vi "MarkerRole.vi"(7 "firstCall":bool, 8 "error in (no error)":errorcluster, 10 "Game in":refnum<class "Game.lvclass">, 11 "MarkerRole in":refnum<class "MarkerRole.lvclass">) -> (0 "error out":errorcluster, 1 "Game out":refnum<class "Game.lvclass">, 2 "Robot out":refnum<class "Robot.lvclass">, 3 "MarkerRole out":refnum<class "MarkerRole.lvclass">)   [LabVIEW 2020, in "MarkerRole.lvclass"]
uses:
  MarkerRole.lvclass
  Tacticbook_class/Tacticbook.lvclass
  MarkerTactic_class/MarkerTactic.lvclass
  MarkerTactic_class/MarkerTacticStates.ctl
  Game_class/Game.lvclass
  Robot_class/Robot.lvclass
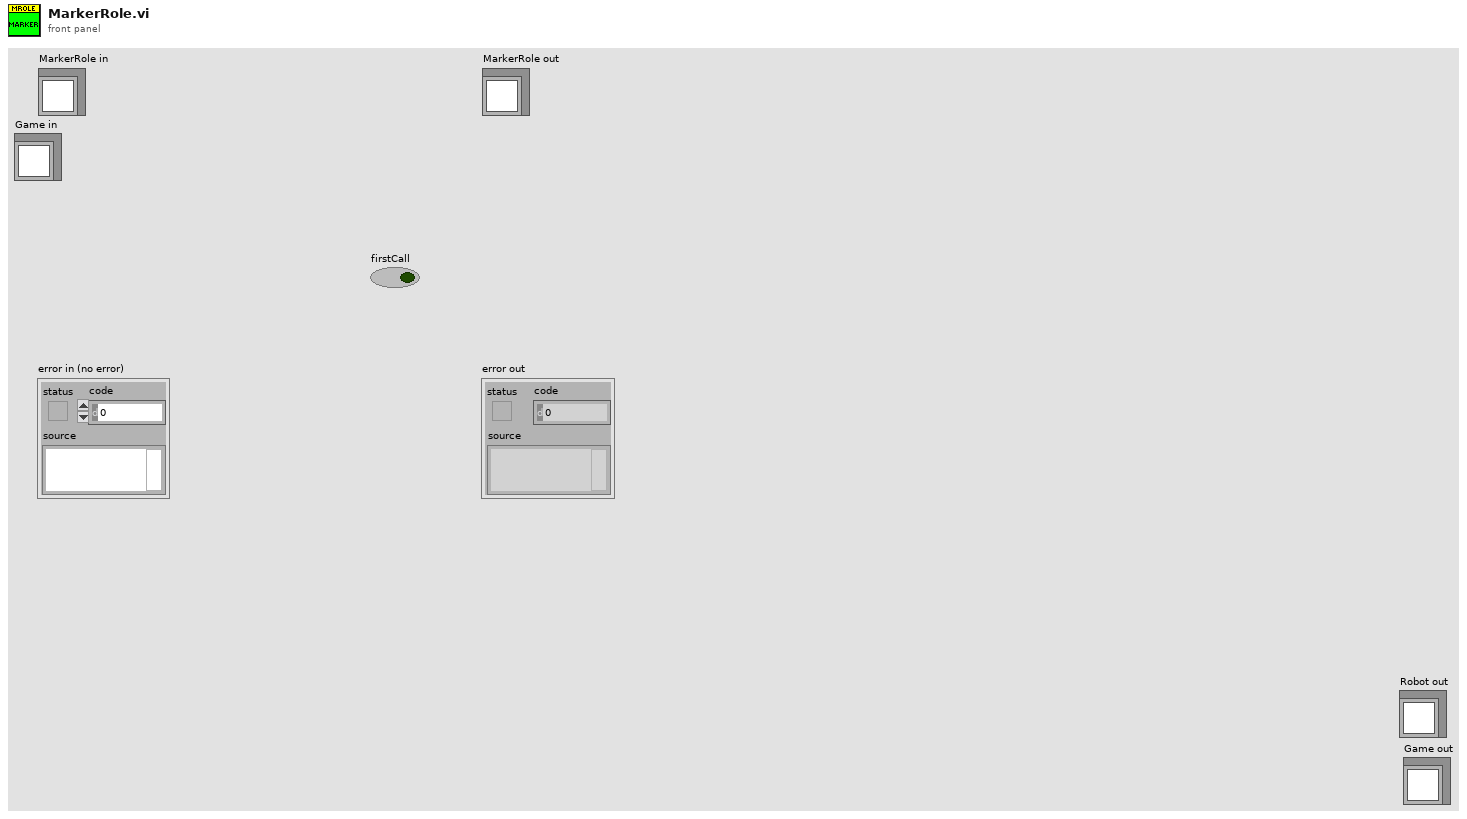
[diagram p1: front panel]
types:
  T1 = typedef "MarkerTacticStates.ctl" = enum16{"Exit", "BlockOurGoal", "FollowAttacker", "BlockEnemyPass"}
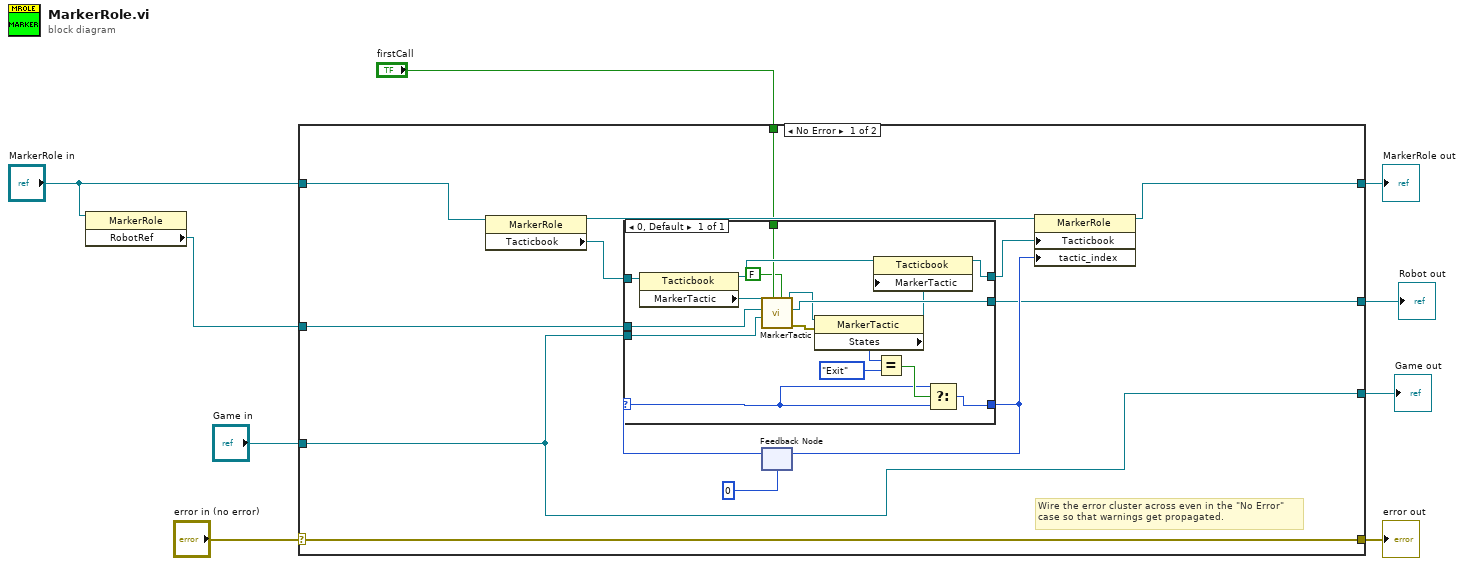
[diagram p0: block diagram]
diagram:
  n1 = property class="MarkerRole"(reference="MarkerRole in") -> ("RobotRef"=w2:refnum<class "Robot.lvclass">)  [unwired: 1 in, 2 out]
  n2 = case shown="No Error" "error in (no error)" {
    selector: "error in (no error)" -> [w22 w42]
    tunnel: [w22 w42] -> w8
    tunnel: [w14 w41] -> w7
    tunnel: "MarkerRole in" -> [w15 w41]
    tunnel: "Game in" -> [w12 w40]
    tunnel: [w13 _] -> w4
    tunnel: [w12 w40] -> w3
    tunnel: w2 -> [w11 _]
    tunnel: "firstCall" -> [w10 _]
    frame No Error {
      # "Wire the error cluster across even in the \"No Error\"\ncase so that warnings get propagated."
      n3 = property class="MarkerRole"(reference=w15) -> (reference out=w21:refnum<class "MarkerRole.lvclass">, "Tacticbook"=w18:refnum<class "Tacticbook.lvclass">)  [unwired: 1 in, 1 out]
      n4 = feedback #1(0) -> (w19:i32)
      n5 = case shown="0, Default" w19 {
        selector: w19 -> [w26]
        tunnel: [w32] -> w17
        tunnel: w18 -> [w39]
        tunnel: [w37] -> w13
        tunnel: [w29] -> w16
        tunnel: w12 -> [w28]
        tunnel: w11 -> [w27]
        tunnel: w10 -> [w24]
        frame 0, Default {
          n6 = property class="Tacticbook"(reference=w39) -> (reference out=w31:refnum<class "Tacticbook.lvclass">, "MarkerTactic"=w38:refnum<class "MarkerTactic.lvclass">)  [unwired: 1 in, 1 out]
          n7 = call-dynamic "MarkerTactic.vi"("SecondMostDangerous"=FALSE, "firstCall"=w24, "Game in"=w28, "Robot"=w27, "MarkerTactic in"=w38) -> ("error out"=w36:errorcluster, "Robot out"=w37:refnum<class "Robot.lvclass">, "MarkerTactic out"=w35:refnum<class "MarkerTactic.lvclass">)  [unwired: 4 in]
          n8 = property class="MarkerTactic"(reference=w35, error in=w36) -> (reference out=w30:refnum<class "MarkerTactic.lvclass">, "States"=w34:T1)  [unwired: 1 out]
          n9 = property class="Tacticbook"(reference=w31, "MarkerTactic"=w30) -> (reference out=w29:refnum<class "Tacticbook.lvclass">)  [unwired: 1 in, 1 out]
          n10 = Equal?(x=w34, y=MarkerTacticStates."Exit") -> (x = y?=w33:bool)
          n11 = Select(t=w26, s=w33, f=w26) -> (s? t:f=w32:i32)
        }
      }
      n12 = feedback-in #1(w17) -> ()
      n13 = property class="MarkerRole"(reference=w21, "Tacticbook"=w16, "tactic_index"=w17) -> (reference out=w14:refnum<class "MarkerRole.lvclass">)  [unwired: 1 in, 1 out]
    }
    frame Error {
    }
  }
  "error out" <- w8
  "MarkerRole out" <- w7
  "Robot out" <- w4
  "Game out" <- w3
